vi "Convert Acceleration to Device Units.vi"(9 "Microstep Size (0)":dbl, 10 "Units (0: device acceleration units)":u16(ring) items=["device acceleration units", "microns per second squared", "millimeters per second squared", "inches per second squared", "degrees per second squared"], 11 "Acceleration (0)":dbl) -> (1 "Device Acceleration (64-bit)":i64, 2 "Device Acceleration (String)":string, 3 "Device Acceleration (32-bit)":i32)   [LabVIEW 2018, in "Zaber A Series.lvlib"]
doc: "Helper to convert standard units of acceleration to device-specific acceleration units.\n\nSelect a unit to convert from and enter an Acceleration quantity. \n\nIf you select a unit other than device units, you must also provide the Microstep Size conversion factor from microsteps to micrometers (for linear devices) or degrees (for rotary devices), which can be found in your device manual."
uses:
  Zaber A Series.lvlib
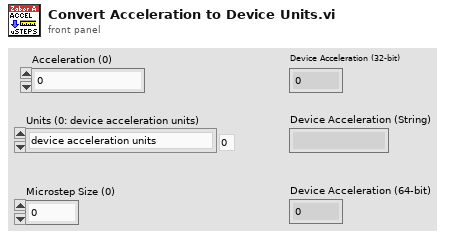
[diagram p1: front panel]
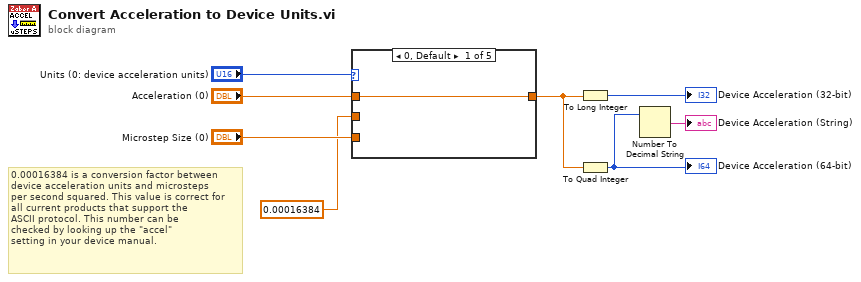
[diagram p0: block diagram]
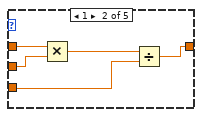
[diagram p2: hidden frame]
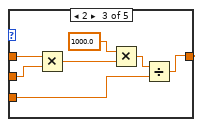
[diagram p3: hidden frame]
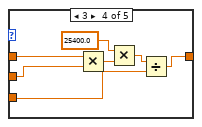
[diagram p4: hidden frame]
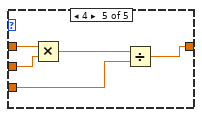
[diagram p5: hidden frame]
diagram:
  # "0.00016384 is a conversion factor between \ndevice acceleration units and microsteps \nper second squared. This value is correct for\nall current products that support the\nASCII protocol. This number can be \nchecked by looking up the \"accel\"\nsetting in your device manual."
  n1 = case shown="0, Default" "Units (0: device acceleration units)" {
    tunnel: 0.00016384 ("Acceleration Constant (0.00016384)") -> [_ w13 w18 w27 w30]
    tunnel: "Microstep Size (0)" -> [_ w12 w17 w26 w29]
    tunnel: "Acceleration (0)" -> [w9 w14 w19 w28 w31]
    tunnel: [w9 w11 w15 w25 w32] -> w1
    frame 0, Default {
    }
    frame 1 {
      n2 = Multiply(x=w14, y=w13) -> (x*y=w10:dbl)
      n3 = Divide(x=w10, y=w12) -> (x/y=w11:dbl)
    }
    frame 2 {
      n4 = Multiply(x=w19, y=w18) -> (x*y=w16:dbl)
      n5 = Multiply(x=1000.0, y=w16) -> (x*y=w21:dbl)
      n6 = Divide(x=w21, y=w17) -> (x/y=w15:dbl)
    }
    frame 3 {
      n7 = Multiply(x=w28, y=w27) -> (x*y=w23:dbl)
      n8 = Multiply(x=25400.0, y=w23) -> (x*y=w22:dbl)
      n9 = Divide(x=w22, y=w26) -> (x/y=w25:dbl)
    }
    frame 4 {
      n10 = Multiply(x=w31, y=w30) -> (x*y=w33:dbl)
      n11 = Divide(x=w33, y=w29) -> (x/y=w32:dbl)
    }
  }
  n12 = To Long Integer(number=w1) -> (32bit integer=→"Device Acceleration (32-bit)":i32)
  n13 = To Quad Integer(1:w1) -> (0:w2:i64)
  "Device Acceleration (64-bit)" <- w2
  n14 = Number To Decimal String(number=w2) -> (decimal integer string=→"Device Acceleration (String)":string)  [unwired: 1 in]
